vi "HandlePythonMessage.vi"(8 "error in (no error)":errorcluster, 10 "Call in":refnum<class "Call.lvclass">, 11 "Node in":refnum<class "CallHandler.lvclass">) -> (0 "error out":errorcluster, 2 "Response Data":variant, 3 "Node out":refnum<class "CallHandler.lvclass">)   [LabVIEW 2013, in "JKI_Python_Bridge_for_LV.lvlib" / "CallHandler.lvclass"]
uses:
  CallHandler.lvclass
  Call/Call.lvclass
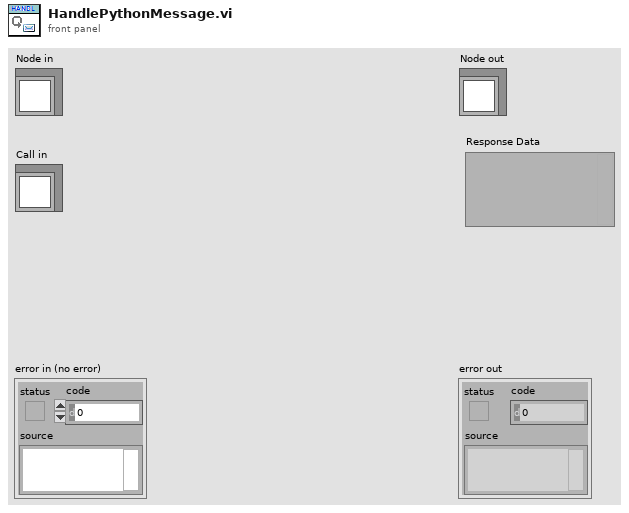
[diagram p1: front panel]
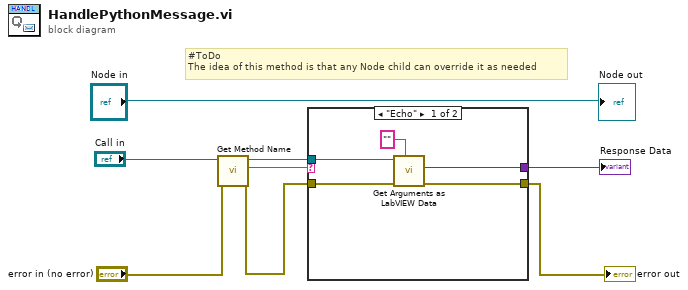
[diagram p0: block diagram]
diagram:
  # "#ToDo\nThe idea of this method is that any Node child can override it as needed"
  n1 = call "Get Method Name.vi"("error in (no error)"="error in (no error)", "Call in"="Call in") -> ("error out"=w3:errorcluster, "Object Name"=w5:string, "Call out"=w4:refnum<class "Call.lvclass">)  [unwired: 6 in, 1 out]
  n2 = case shown="\"Echo\"" w5 {
    tunnel: w4 -> [w12 _]
    tunnel: w3 -> [w11 w14]
    tunnel: [w10 w14] -> w2
    tunnel: [w9 _] -> w1
    frame "Echo" {
      n3 = call "Get Arguments as LabVIEW Data.vi"("type"="", "error in (no error)"=w11, "Call in"=w12) -> ("error out"=w10:errorcluster, "LabVIEW Data"=w9:variant)  [unwired: 6 in, 1 out]
    }
    frame Default {
    }
  }
  "error out" <- w2
  "Response Data" <- w1
  "Node out" <- "Node in"
